vi "非断电保持全局变量.vi"() -> ()   [LabVIEW 2016]
panel:
  in  "数据库类型":T1
  in  "Password":string="783523103"
  in  "站点名称":string
  in  "权限等级":enum16{"一级权限", "二级权限", "三级权限", "超级权限"}(ring)
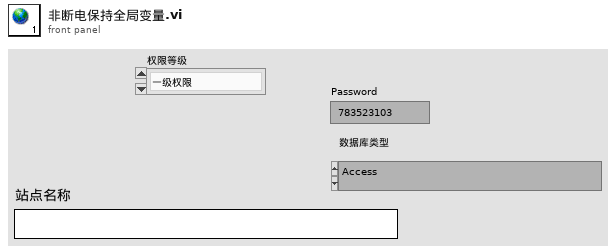
[diagram p1: front panel]
types:
  T1 = typedef "数据库类型.ctl" = enum16{"Access", "SQLite"}
diagram:
